vi "Get LS Data.vi"(8 "Initial LS Data":T1={"Total Cycles"=[0, 0, 0, 0, 0, 0], "Steps"=[0, 0, 0, 0, 0, 0], "Anomalies Total"=[0, 0, 0, 0, 0, 0], "Cycles"=[0, 0, 0, 0, 0, 0], "Anomalies/Cycle"=[0, 0, 0, 0, 0, 0], "Anomalies (Last Cycle)"=[0, 0, 0, 0, 0, 0], "Opens"=[0, 0, 0, 0, 0, 0]} {"Opens" format="%#.0f"; "Anomalies (Last Cycle)" format="%#.0f"; "Anomalies/Cycle" format="%#.0f"; "Cycles" format="%#.0f"; "Anomalies Total" format="%#.0f"; "Steps" format="%#.0f"; "Total Cycles" format="%#.0f"}, 11 "FPGA Ref":T2) -> (3 "LS Data":T1 {"Opens" format="%#.0f"; "Anomalies (Last Cycle)" format="%#.0f"; "Anomalies/Cycle" format="%#.0f"; "Cycles" format="%#.0f"; "Anomalies Total" format="%#.0f"; "Steps" format="%#.0f"; "Total Cycles" format="%#.0f"})   [LabVIEW 2019]
uses:
  Controls/FPGA_Reference.ctl
  Type Defs/LS Data.ctl
  <vilib>/Utility/error.llb/Error Cluster From Error Code.vi
  <vilib>/rvi/errors/niLvFpgaAdjustHostInterfaceError.vi
  <vilib>/rvi/interface/nirviReadWriteControl/nirviReadWriteControl.xnode
  FPGA Bitfiles/LS_Durability_FPGA_9627.lvbitx
  NiFpgaLv.dll
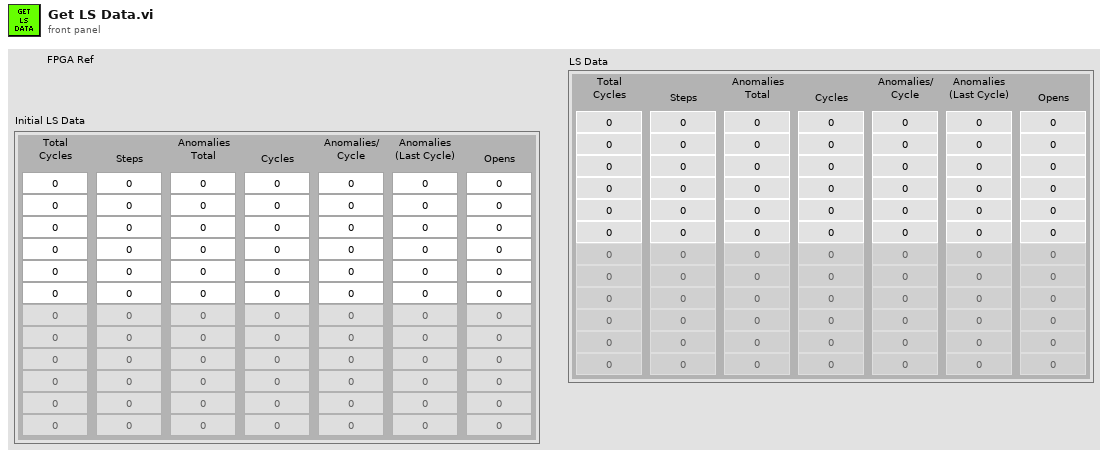
[diagram p1: front panel]
types:
  T1 = typedef "LS Data.ctl" = cluster{"Total Cycles":u32[], "Steps":u32[], "Anomalies Total":i32[], "Cycles":u32[], "Anomalies/Cycle":i32[], "Anomalies (Last Cycle)":i32[], "Opens":i32[]}
  T2 = typedef "FPGA_Reference.ctl" = refnum<k20>
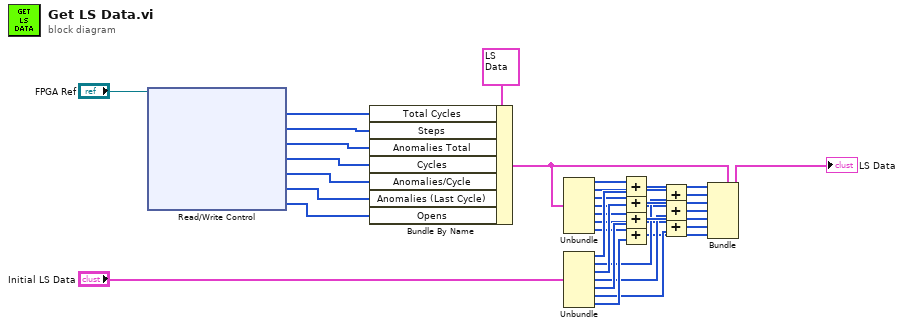
[diagram p0: block diagram]
diagram:
  n1 = xnode "Read/Write Control"("FPGA VI Reference In"="FPGA Ref") -> ("Total Cycles"=w31:u32[], "Steps"=w30:u32[], "Anomalies (Total)"=w29:i32[], "Cycles"=w28:u32[], "Anomalies/Cycle"=w27:i32[], "Anomalies (Last Cycle)"=w26:i32[], "Opens Detected"=w25:u16[])  [unwired: 1 in, 2 out]
  n2 = Bundle By Name(cluster=T1 {"Total Cycles"=[0, 0, 0, 0, 0, 0, 0, 0, 0, 0, 0, 0], "Steps"=[0, 0, 0, 0, 0, 0, 0, 0, 0, 0, 0, 0], "Anomalies Total"=[0, 0, 0, 0, 0, 0, 0, 0, 0, 0, 0, 0], "Cycles"=[0, 0, 0, 0, 0, 0, 0, 0, 0, 0, 0, 0], "Anomalies/Cycle"=[0, 0, 0, 0, 0, 0, 0, 0, 0, 0, 0, 0], "Anomalies (Last Cycle)"=[0, 0, 0, 0, 0, 0, 0, 0, 0, 0, 0, 0], "Opens"=[]} ("LS Data"), "Total Cycles"=w31, "Steps"=w30, "Anomalies Total"=w29, "Cycles"=w28, "Anomalies/Cycle"=w27, "Anomalies (Last Cycle)"=w26, "Opens"=w25) -> (w4:T1)
  n3 = Unbundle(w4) -> ("Total Cycles"=w5:u32[], "Steps"=w6:u32[], "Anomalies Total"=w7:i32[], "Cycles"=w8:u32[], "Anomalies/Cycle"=w9:i32[], "Anomalies (Last Cycle)"=w10:i32[], "Opens"=w11:i32[])
  n4 = Unbundle("Initial LS Data") -> ("Total Cycles"=w12:u32[], "Steps"=w13:u32[], "Anomalies Total"=w14:i32[], "Cycles"=w15:u32[], "Anomalies/Cycle"=w16:i32[], "Anomalies (Last Cycle)"=w17:i32[], "Opens"=w18:i32[])
  n5 = Add(x=w5, y=w12) -> (x+y=w19:u32[])
  n6 = Add(x=w7, y=w14) -> (x+y=w21:i32[])
  n7 = Add(x=w9, y=w16) -> (x+y=w23:i32[])
  n8 = Add(x=w11, y=w18) -> (x+y=w1:i32[])
  n9 = Add(x=w6, y=w13) -> (x+y=w20:u32[])
  n10 = Add(x=w8, y=w15) -> (x+y=w22:u32[])
  n11 = Add(x=w10, y=w17) -> (x+y=w24:i32[])
  n12 = Bundle(cluster=w4, "Total Cycles"=w19, "Steps"=w20, "Anomalies Total"=w21, "Cycles"=w22, "Anomalies/Cycle"=w23, "Anomalies (Last Cycle)"=w24, "Opens"=w1) -> (→"LS Data":T1)
